vi "S2C_M2p5942_Proc_Clock.vi"(7 "Local?":bool, 8 "Error In":errorcluster, 10 "Command":string, 11 "JSON String":string) -> (0 "Error Out":errorcluster, 3 "Response":variant)   [LabVIEW 2024]
uses:
  S2C_M2p5942_Proc_Globals.vi
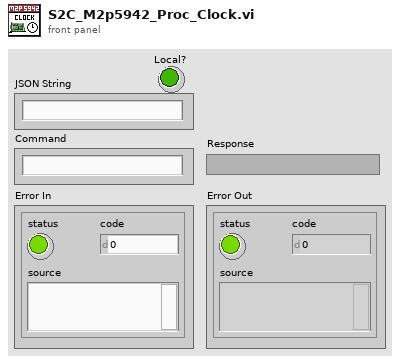
[diagram p1: front panel]
types:
  T1 = cluster{"Clock Mode":u16, "Sampling Rate (kHz)":dbl, "Clock Output":bool, "Termination":bool, "Ref. Clock (MHz)":dbl, "Threshold (mV)":i32}
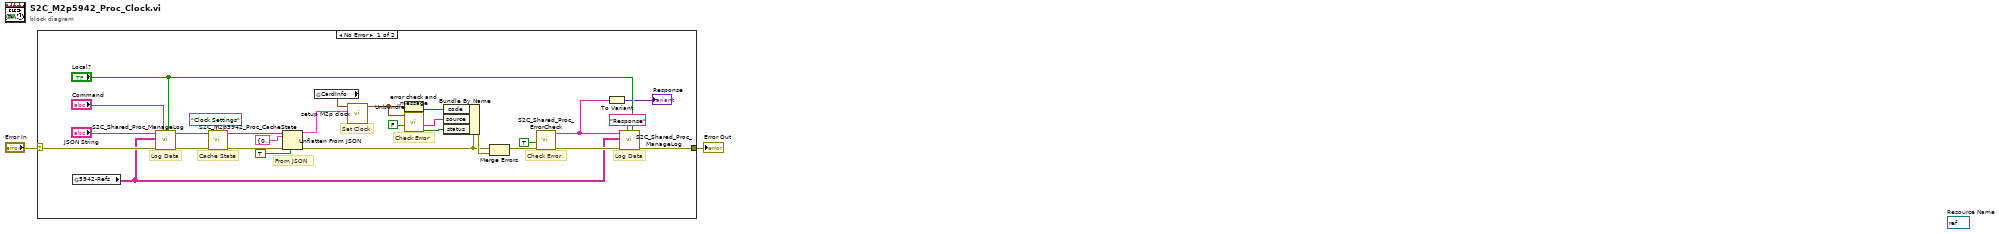
[diagram p0: block diagram]
diagram:
  (unwired) refnum<visa-resource-name> refnum  # Resource Name
  n1 = case shown="No Error" "Error In" {
    selector: "Error In" -> [w29 w31]
    tunnel: [w27 w31] -> w1
    frame No Error {
      # "Check Error"
      # "Set Clock"
      # "Check Error"
      # "Cache State"
      # "Log Data"
      # "Log Data"
      # "From JSON"
      n2 = global read "S2C_M2p5942_Proc_Globals.vi" "5942-Refs"() -> (w17:string[][])
      n3 = call "S2C_Shared_Proc_ManageLog.vi"("Local?"="Local?", "Command"="Command", "Error In"=w29, "Refs"=w17, "Data In"="JSON String") -> ("Error Out"=w25:errorcluster, "Data Out"=w24:string)  [unwired: 5 in]
      n4 = call "S2C_M2p5942_Proc_CacheState.vi"("Label"="Clock Settings", "Error In"=w25, "Data In"=w24) -> ("Error Out"=w22:errorcluster, "Data Out"=w23:string)  [unwired: 7 in]
      n5 = Unflatten From JSON(JSON string=w23, type and defaults=T1 {"Clock Mode"=0, "Sampling Rate (kHz)"=10000.0, "Clock Output"=TRUE, "Termination"=TRUE, "Ref. Clock (MHz)"=10.0, "Threshold (mV)"=1500} ("Clock Settings"), default null elements? (F)=TRUE, error in (no error)=w22) -> (value=w11:T1, error out=w5:errorcluster)  [unwired: 3 in]
      n6 = global read "S2C_M2p5942_Proc_Globals.vi" "CardInfo"() -> (w13:cluster{"Card Handle":u64, "Error Code":u32})
      n7 = call "setup M2p clock.vi"("Clock Settings"=w11, "Card Info In"=w13) -> ("Card Info Out"=w4:cluster{"Card Handle":u64, "Error Code":u32})  [unwired: 4 in, 1 out]
      n8 = Unbundle(w4) -> ("Error Code"=w8:u32)  [unwired: 1 out]
      n9 = call "error check and message.vi"("Display Message (true)"=FALSE, "Card Info In"=w4) -> ("Error occurred"=w6:bool, "Error Message"=w7:string)  [unwired: 3 in, 1 out]
      n10 = Bundle By Name(cluster=w5, "code"=w8, "source"=w7, "status"=w6) -> (w10:errorcluster)
      n11 = Merge Errors(w5, w10) -> (w3:errorcluster)
      n12 = call "S2C_Shared_Proc_ErrorCheck.vi"("Error In"=w3, "ExpReply?"=TRUE) -> ("Error Out"=w19:errorcluster, "Status"=w15:string)  [unwired: 8 in]
      n13 = To Variant(anything=w15) -> (Variant=→"Response":variant)
      n14 = call "S2C_Shared_Proc_ManageLog.vi"("Local?"="Local?", "Command"="Response", "Error In"=w19, "Refs"=w17, "Data In"=w15) -> ("Error Out"=w27:errorcluster)  [unwired: 5 in, 1 out]
    }
    frame Error {
    }
  }
  "Error Out" <- w1
